vi "N-PCI6221-V02.vi"(8 "error in":errorcluster caption="错误输入", 9 "L":string, 10 "H":string, 11 "Input":string) -> (0 "error out":errorcluster caption="错误输出", 2 "布尔":bool, 3 "Output":string)   [LabVIEW 2014]
uses:
  <vilib>/DAQmx/create/channels.llb/DAQmx Create Channel (DO-Digital Output).vi
  <vilib>/DAQmx/write.llb/DAQmx Write (Digital 1D Bool 1Chan 1Samp).vi
  <vilib>/DAQmx/create/channels.llb/DAQmx Create Channel (DI-Digital Input).vi
  <vilib>/DAQmx/read.llb/DAQmx Read (Digital U8 1Chan 1Samp).vi
  <vilib>/DAQmx/read.llb/DAQmx Read (Digital Bool 1Line 1Point).vi
  <vilib>/DAQmx/write.llb/DAQmx Write (Digital 1D Bool NChan 1Samp 1Line).vi
  <vilib>/DAQmx/create/channels.llb/DAQmx Create Channel (AI-Voltage-Basic).vi
  <vilib>/DAQmx/read.llb/DAQmx Read (Analog 1D DBL 1Chan NSamp).vi
  <vilib>/DAQmx/read.llb/DAQmx Read (Analog DBL 1Chan 1Samp).vi
  <vilib>/DAQmx/configure/timing.llb/DAQmx Timing (Sample Clock).vi
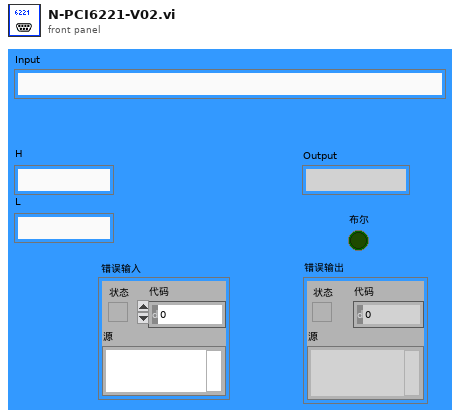
[diagram p1: front panel]
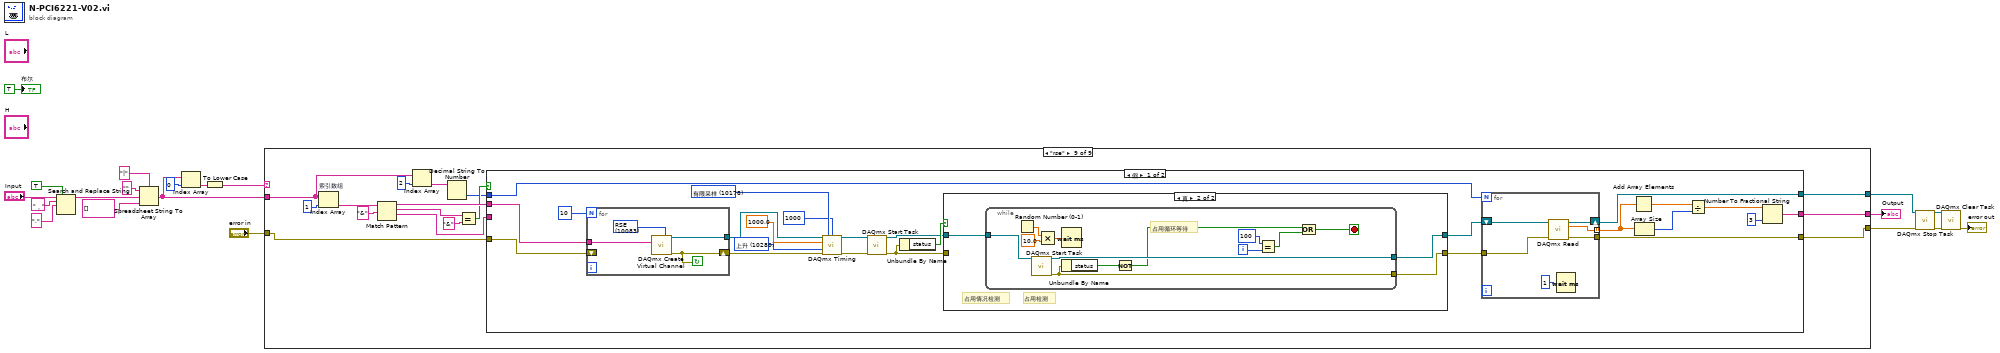
[diagram p0: block diagram]
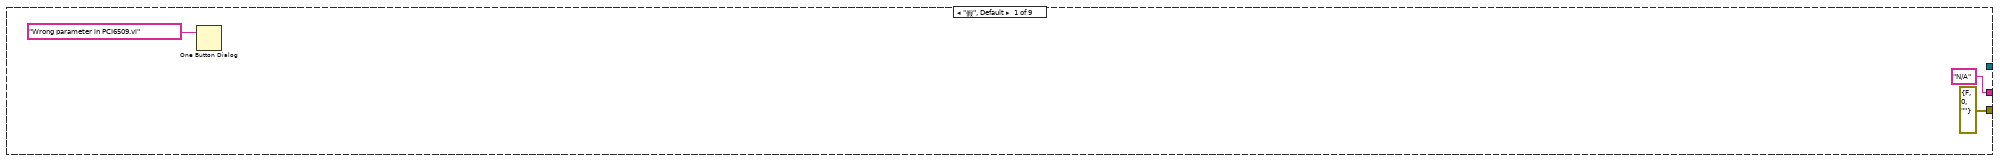
[diagram p2: hidden frame]
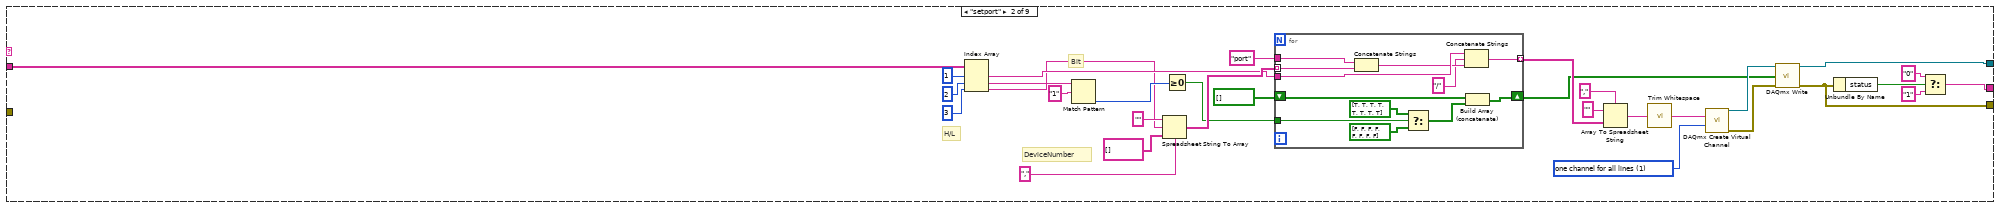
[diagram p3: hidden frame]
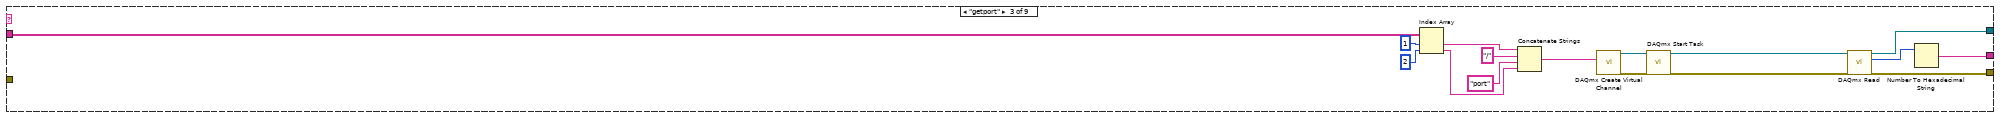
[diagram p4: hidden frame]
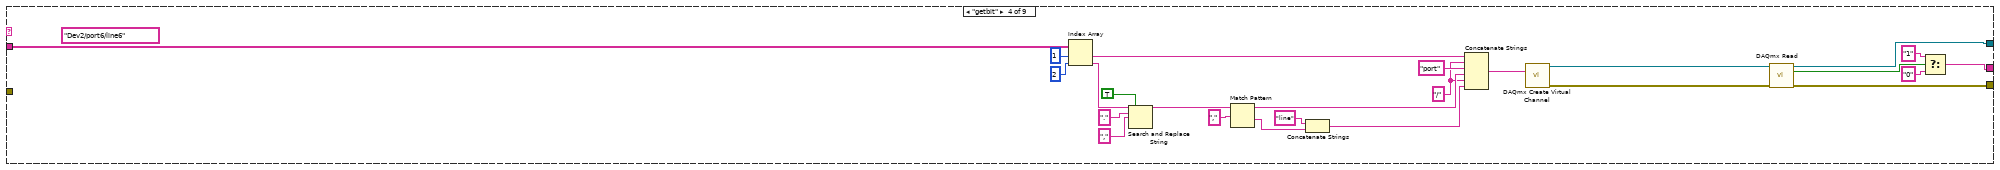
[diagram p5: hidden frame]
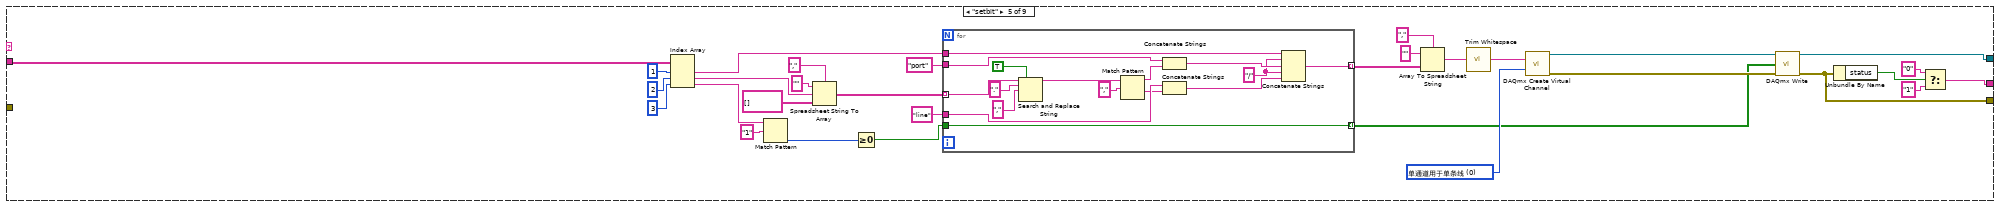
[diagram p6: hidden frame]
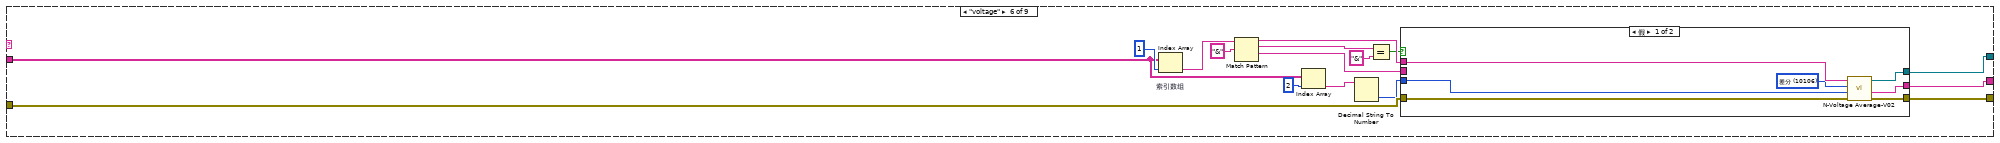
[diagram p7: hidden frame]
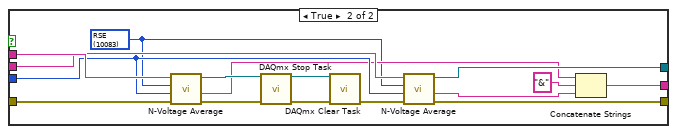
[diagram p8: hidden frame]
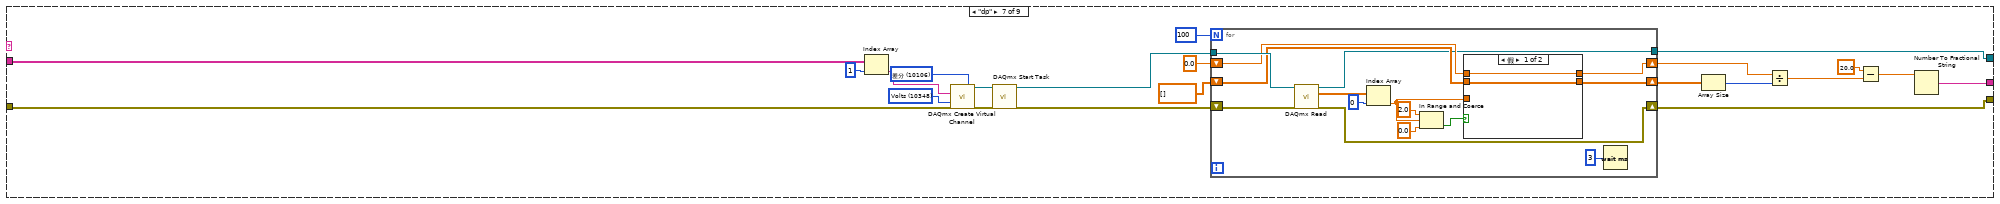
[diagram p9: hidden frame]
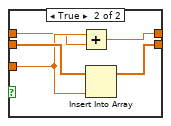
[diagram p10: hidden frame]
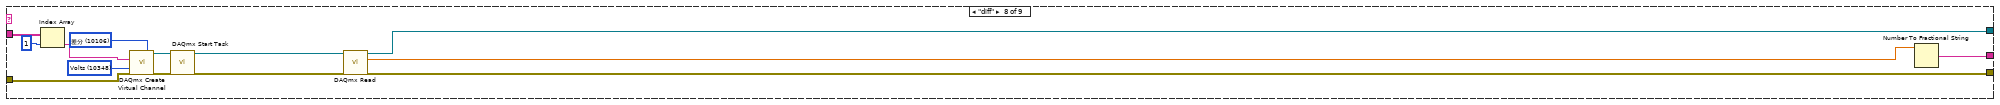
[diagram p11: hidden frame]
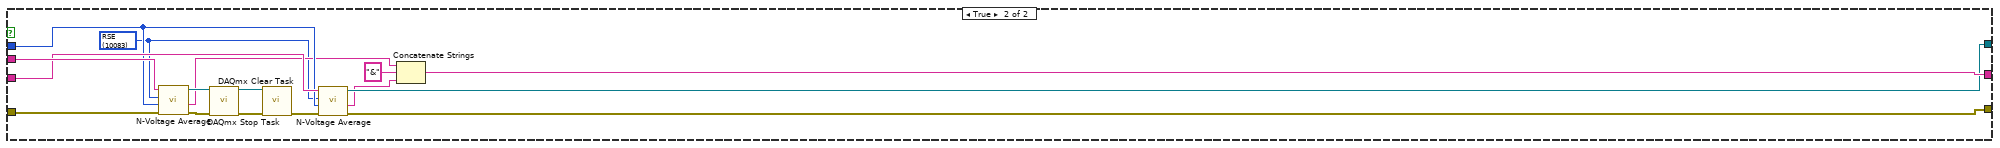
[diagram p13: hidden frame]
diagram:
  n1 = Search and Replace String(replace all?=TRUE ("替换全部？(F)"), input string="Input", search string="，" ("搜索字符串"), replace string="," ("替换字符串(\"\")")) -> (result string=w4:string)  [unwired: 4 in, 3 out]
  n2 = Spreadsheet String To Array(delimiter (Tab)="|" ("分隔符(Tab)"), format string="" ("格式字符串"), spreadsheet string=w4, array type (2D Dbl)=string[] []) -> (array=w2:string[])
  n3 = Index Array(array=w2, index=0 ("索引")) -> (element=w16:string)
  n4 = To Lower Case(string=w16) -> (all lower case string=w15:string)
  n5 = case shown="\"rse\"" w15 {
    tunnel: w2 -> [_ w31 w70 w87 w138 w157 w210 w246 w256]
    tunnel: [_ w29 w67 w85 w115 w168 w199 w241 w253] -> w14
    tunnel: [errorcluster {"status"=FALSE, "code"=0, "source"=""} ("error out") w28 w68 w86 w114 w169 w200 w242 w254] -> w13
    tunnel: ["N/A" w24 w69 w84 w110 w166 w201 w243 w255] -> w9
    tunnel: "error in" -> [_ _ _ _ _ w170 w197 w239 w257]
    frame "假", Default {
      n6 = One Button Dialog(message="Wrong parameter in PCI6509.vi") -> ()  [unwired: 2 out]
    }
    frame "setport" {
      w49 = 1 items=["one channel for each line", "one channel for all lines"] ("line grouping")
      # "H/L"
      # "Bit"
      # "DeviceNumber"
      n7 = Index Array(array=w31, index #1=1 ("index"), index #2=2 ("index"), index #3=3 ("index")) -> (element #1=w41:string, element #2=w30:string, element #3=w40:string)
      n8 = Match Pattern(string=w40, regular expression="1") -> (offset past match=w48:i32)  [unwired: 4 out]
      n9 = Spreadsheet String To Array(delimiter (Tab)=",", format string="", spreadsheet string=w30, array type (2D Dbl)=string[] []) -> (array=w45:string[])
      n10 = Greater Or Equal To 0?(x=w48) -> (x >= 0?=w35:bool)
      n11 = for {
        tunnel: w45 -> [w61] mode=indexing
        tunnel: w41 -> [w66]
        tunnel: "port" ("delimiter (Tab)") -> [w65]
        tunnel: [w62] -> w36 mode=indexing
        tunnel: w35 -> [w60]
        shift-right: [w55] -> w33
        shift-left: bool[] [] -> [w57]
        n12 = Concatenate Strings(w65, w61) -> (w64:string)
        n13 = Select(t=bool[] [TRUE, TRUE, TRUE, TRUE, TRUE, TRUE, TRUE, TRUE], s=w60, f=bool[] [FALSE, FALSE, FALSE, FALSE, FALSE, FALSE, FALSE, FALSE]) -> (s? t:f=w56:bool[])
        n14 = Concatenate Strings(w66, "/" ("delimiter (Tab)"), w64) -> (w62:string)
        n15 = Build Array (concatenate)(w57, w56) -> (w55:bool[])
      }
      n16 = Array To Spreadsheet String(delimiter (Tab)=",", array=w36, 3:"" ("format string")) -> (spreadsheet string=w37:string)
      n17 = call <vilib>:"Trim Whitespace.vi"("string"=w37) -> ("trimmed string"=w32:string)  [unwired: 1 in]
      n18 = call-poly <vilib>:"DAQmx Create Virtual Channel.vi"("lines"=w32, "line grouping"=w49) -> ("task out"=w50:refnum<k21>, "error out"=w51:errorcluster)  [unwired: 3 in, 9 out]
      n19 = call-poly <vilib>:"DAQmx Write.vi"("task/channels in"=w50, "data"=w33, "error in"=w51) -> ("task out"=w29:refnum<k21>, "error out"=w28:errorcluster)  [unwired: 1 in, 10 out]
      n20 = Unbundle By Name(w28) -> ("status"=w27:bool)
      n21 = Select(t="0", s=w27, f="1") -> (s? t:f=w24:string)
    }
    frame "getport" {
      n22 = Index Array(array=w70, index #1=1 ("index"), index #2=2 ("index")) -> (element #1=w80:string, element #2=w77:string)
      n23 = Concatenate Strings(w80, "/" ("string"), "port" ("string"), w77) -> (w76:string)
      n24 = call-poly <vilib>:"DAQmx Create Virtual Channel.vi"("lines"=w76) -> ("task out"=w74:refnum<k21>, "error out"=w71:errorcluster)  [unwired: 4 in, 9 out]
      n25 = call <vilib>:"DAQmx Start Task.vi"("task/channels in"=w74, "error in"=w71) -> ("task out"=w73:refnum<k21>, "error out"=w72:errorcluster)  [unwired: 12 out]
      n26 = call-poly <vilib>:"DAQmx Read.vi"("task/channels in"=w73, "error in"=w72) -> ("task out"=w67:refnum<k21>, "data"=w75:u8, "error out"=w68:errorcluster)  [unwired: 11 out]
      n27 = Number To Hexadecimal String(2:w75) -> (0:w69:string)  [unwired: 1 out]
    }
    frame "getbit" {
      (unwired) tag "Dev2/port6/line6" ("lines")
      w94 = "/" ("string")
      n28 = Index Array(array=w87, index #1=1 ("index"), index #2=2 ("index")) -> (element #1=w103:string, element #2=w100:string)
      n29 = Search and Replace String(replace all?=TRUE ("replace all? (F)"), input string=w100, search string=".", replace string="," ("replace string (\"\")")) -> (result string=w97:string)  [unwired: 1 in, 6 out]
      n30 = Match Pattern(string=w97, regular expression=",") -> (before substring=w95:string, after substring=w92:string)  [unwired: 3 out]
      n31 = Concatenate Strings("line" ("string"), w92) -> (w91:string)
      n32 = Concatenate Strings(w103, w94, "port" ("string"), w95, w94, w91) -> (w90:string)
      n33 = call-poly <vilib>:"DAQmx Create Virtual Channel.vi"("lines"=w90) -> ("task out"=w105:refnum<k21>, "error out"=w104:errorcluster)  [unwired: 4 in, 9 out]
      n34 = call-poly <vilib>:"DAQmx Read.vi"("task/channels in"=w105, "error in"=w104) -> ("task out"=w85:refnum<k21>, "data"=w83:bool, "error out"=w86:errorcluster)  [unwired: 11 out]
      n35 = Select(t="1", s=w83, f="0") -> (s? t:f=w84:string)
    }
    frame "setbit" {
      w119 = 0 items=["单通道用于单条线", "单通道用于所有线"] ("line grouping")
      n36 = Index Array(array=w138, index #1=1 ("索引"), index #2=2 ("索引"), index #3=3 ("索引")) -> (element #1=w129:string, element #2=w135:string, element #3=w126:string)
      n37 = Match Pattern(string=w126, regular expression="1" ("正则表达式")) -> (offset past match=w124:i32)  [unwired: 4 out]
      n38 = Spreadsheet String To Array(delimiter (Tab)="," ("分隔符(Tab)"), format string="" ("格式字符串"), spreadsheet string=w135, array type (2D Dbl)=string[] []) -> (array=w128:string[])
      n39 = Greater Or Equal To 0?(x=w124) -> (x >= 0?=w123:bool)
      n40 = for {
        tunnel: w128 -> [w141] mode=indexing
        tunnel: w129 -> [w153]
        tunnel: "port" ("格式字符串") -> [w152]
        tunnel: "line" ("格式字符串") -> [w150]
        tunnel: [w145] -> w122 mode=indexing
        tunnel: w123 -> [w139]
        tunnel: [w139] -> w116 mode=indexing
        w147 = "/" ("delimiter (Tab)")
        n41 = Search and Replace String(replace all?=TRUE ("replace all? (F)"), input string=w141, search string=".", replace string="," ("replace string (\"\")")) -> (result string=w140:string)  [unwired: 1 in, 6 out]
        n42 = Match Pattern(string=w140, regular expression=",") -> (before substring=w151:string, after substring=w149:string)  [unwired: 3 out]
        n43 = Concatenate Strings(w152, w151) -> (w148:string)
        n44 = Concatenate Strings(w150, w149) -> (w146:string)
        n45 = Concatenate Strings(w153, w147, w148, w147, w146) -> (w145:string)
      }
      n46 = Array To Spreadsheet String(delimiter (Tab)="," ("分隔符(Tab)"), array=w122, 3:"" ("格式字符串")) -> (spreadsheet string=w109:string)
      n47 = call <vilib>:"Trim Whitespace.vi"("string"=w109) -> ("trimmed string"=w108:string)  [unwired: 1 in]
      n48 = call-poly <vilib>:"DAQmx Create Virtual Channel.vi"("lines"=w108, "line grouping"=w119) -> ("task out"=w118:refnum<k21>, "error out"=w117:errorcluster)  [unwired: 3 in, 9 out]
      n49 = call-poly <vilib>:"DAQmx Write.vi"("task/channels in"=w118, "data"=w116, "error in"=w117) -> ("task out"=w115:refnum<k21>, "error out"=w114:errorcluster)  [unwired: 1 in, 10 out]
      n50 = Unbundle By Name(w114) -> ("status"=w113:bool)
      n51 = Select(t="0", s=w113, f="1") -> (s? t:f=w110:string)
    }
    frame "voltage" {
      n52 = Index Array "索引数组"(array=w157, index=1) -> (element=w165:string)
      n53 = Match Pattern(string=w165, regular expression="&" ("正则表达式")) -> (before substring=w161:string, match substring=w163:string, after substring=w160:string)  [unwired: 1 in, 1 out]
      n54 = Index Array(array=w157, index=2) -> (element=w156:string)
      n55 = Decimal String To Number(string=w156) -> (number=w155:i32)  [unwired: 2 in, 1 out]
      n56 = Equal?(x=w163, y="&" ("正则表达式")) -> (x = y?=w159:bool)
      n57 = case shown="假" w159 {
        tunnel: w170 -> [w176 w193]
        tunnel: [w175 w183] -> w169
        tunnel: [w174 w182] -> w168
        tunnel: [w173 w184] -> w166
        tunnel: w161 -> [w177 w187]
        tunnel: w160 -> [_ w186]
        tunnel: w155 -> [w172 w181]
        frame False {
          w171 = 10106 items=["默认"=-1, "RSE"=10083, "NRSE"=10078, "差分"=10106, "伪差分"=12529] ("Type")
          n58 = call "N-Voltage Average-V02.vi"("error in"=w176, "Times"=w172, "Type"=w171, "Channel"=w177) -> ("error out"=w175:errorcluster, "Voltage"=w173:string, "task out"=w174:refnum<k21>)  [unwired: 1 in]
        }
        frame True {
          w178 = 10083 items=["默认"=-1, "RSE"=10083, "NRSE"=10078, "差分"=10106, "伪差分"=12529] ("Type")
          n59 = call "N-Voltage Average.vi"("error in"=w193, "Times"=w181, "Type"=w178, "Channel"=w187) -> ("error out"=w189:errorcluster, "Voltage"=w180:string, "task out"=w190:refnum<k21>)  [unwired: 1 in]
          n60 = call <vilib>:"DAQmx Stop Task.vi"("task/channels in"=w190, "error in"=w189) -> ("task out"=w191:refnum<k21>, "error out"=w192:errorcluster)  [unwired: 12 out]
          n61 = call <vilib>:"DAQmx Clear Task.vi"("task in"=w191, "error in"=w192) -> ("error out"=w188:errorcluster)  [unwired: 13 out]
          n62 = call "N-Voltage Average.vi"("error in"=w188, "Times"=w181, "Type"=w178, "Channel"=w186) -> ("error out"=w183:errorcluster, "Voltage"=w179:string, "task out"=w182:refnum<k21>)  [unwired: 1 in]
          n63 = Concatenate Strings(w180, "&" ("字符串"), w179) -> (w184:string)
        }
      }
    }
    frame "dp" {
      w212 = 10348 items=["Volts"=10348, "来自自定义换算"=10065] ("units")
      w215 = 10106 items=["默认"=-1, "RSE"=10083, "NRSE"=10078, "差分"=10106, "伪差分"=12529] ("input terminal configuration")
      n64 = Index Array(array=w210, index=1) -> (element=w209:string)
      n65 = call-poly <vilib>:"DAQmx Create Virtual Channel.vi"("input terminal configuration"=w215, "physical channels"=w209, "units"=w212, "error in"=w197) -> ("task out"=w213:refnum<k21>, "error out"=w214:errorcluster)  [unwired: 5 in, 5 out]
      n66 = call <vilib>:"DAQmx Start Task.vi"("task/channels in"=w213, "error in"=w214) -> ("task out"=w207:refnum<k21>, "error out"=w198:errorcluster)  [unwired: 12 out]
      n67 = for {
        N: 100 -> [_]
        tunnel: w207 -> [w230]
        shift-right: [w222] -> w205
        shift-left: dbl[] [] -> [w224]
        shift-right: [w220] -> w202
        shift-left: 0.0 ("下限") -> [w221]
        tunnel: [w218] -> w199
        shift-right: [w219] -> w200
        shift-left: w198 -> [w217]
        n68 = call-poly <vilib>:"DAQmx Read.vi"("task/channels in"=w230, "error in"=w217) -> ("task out"=w218:refnum<k21>, "data"=w229:dbl[], "error out"=w219:errorcluster)  [unwired: 1 in, 10 out]
        n69 = Index Array(array=w229, index=0 ("索引")) -> (element=w223:dbl)
        n70 = In Range and Coerce(upper limit=2.0 ("上限"), x=w223, lower limit=0.0 ("下限")) -> (In Range?=w225:bool)  [unwired: 1 out]
        n71 = case shown="假" w225 {
          tunnel: w224 -> [w232 w237]
          tunnel: w223 -> [_ w235]
          tunnel: [w232 w236] -> w222
          tunnel: w221 -> [w231 w234]
          tunnel: [w231 w233] -> w220
          frame False {
          }
          frame True {
            n72 = Add(x=w235, y=w234) -> (x+y=w233:dbl)
            n73 = Insert Into Array(array=w237, new element=w235) -> (w236:dbl[])  [unwired: 1 in]
          }
        }
        n74 = Wait (ms)(milliseconds to wait=u32 3 ("等待时间（毫秒）")) -> ()  [unwired: 1 out]
      }
      n75 = Array Size(array=w205) -> (size(s)=w203:i32)
      n76 = Divide(x=w202, y=w203) -> (x/y=w195:dbl)
      n77 = Subtract(x=20.0 ("下限"), y=w195) -> (x-y=w194:dbl)
      n78 = Number To Fractional String(number=w194) -> (F-format string=w201:string)  [unwired: 3 in]
    }
    frame "diff" {
      w248 = 10348 items=["Volts"=10348, "来自自定义换算"=10065] ("units")
      w251 = 10106 items=["默认"=-1, "RSE"=10083, "NRSE"=10078, "差分"=10106, "伪差分"=12529] ("input terminal configuration")
      n79 = Index Array(array=w246, index=1) -> (element=w245:string)
      n80 = call-poly <vilib>:"DAQmx Create Virtual Channel.vi"("input terminal configuration"=w251, "physical channels"=w245, "units"=w248, "error in"=w239) -> ("task out"=w249:refnum<k21>, "error out"=w250:errorcluster)  [unwired: 5 in, 5 out]
      n81 = call <vilib>:"DAQmx Start Task.vi"("task/channels in"=w249, "error in"=w250) -> ("task out"=w244:refnum<k21>, "error out"=w240:errorcluster)  [unwired: 12 out]
      n82 = call-poly <vilib>:"DAQmx Read.vi"("task/channels in"=w244, "error in"=w240) -> ("task out"=w241:refnum<k21>, "data"=w238:dbl, "error out"=w242:errorcluster)  [unwired: 11 out]
      n83 = Number To Fractional String(number=w238) -> (F-format string=w243:string)  [unwired: 3 in]
    }
    frame "rse" {
      n84 = Index Array "索引数组"(array=w256, index=1) -> (element=w252:string)
      n85 = Match Pattern(string=w252, regular expression="&" ("正则表达式")) -> (before substring=w263:string, match substring=w265:string, after substring=w262:string)  [unwired: 1 in, 1 out]
      n86 = Index Array(array=w256, index=2) -> (element=w259:string)
      n87 = Decimal String To Number(string=w259) -> (number=w258:i32)  [unwired: 2 in, 1 out]
      n88 = Equal?(x=w265, y="&" ("正则表达式")) -> (x = y?=w261:bool)
      n89 = case shown="假" w261 {
        tunnel: w257 -> [w291 w335]
        tunnel: [w287 w325] -> w254
        tunnel: [w288 w324] -> w253
        tunnel: [w289 w326] -> w255
        tunnel: w263 -> [w292 w329]
        tunnel: w262 -> [_ w328]
        tunnel: w258 -> [w290 w323]
        frame False {
          w283 = 10178 items=["有限采样"=10178, "连续采样"=10123, "硬件定时单点"=12522] ("sample mode")
          w284 = 10280 items=["上升"=10280, "下降"=10171] ("active edge")
          n90 = for {
            N: 10 -> [_]
            tunnel: w292 -> [w312]
            tunnel: [w311] -> w279
            shift-right: [w310] -> w278
            shift-left: w291 -> [_]
            stop <- w310 continue-if-true
            w313 = 10083 items=["默认"=-1, "RSE"=10083, "NRSE"=10078, "差分"=10106, "伪差分"=12529] ("Type")
            n91 = call-poly <vilib>:"DAQmx Create Virtual Channel.vi"("input terminal configuration"=w313, "physical channels"=w312) -> ("task out"=w311:refnum<k21>, "error out"=w310:errorcluster)  [unwired: 12 in]
          }
          n92 = call-poly <vilib>:"DAQmx Timing.vi"("task/channels in"=w279, "sample mode"=w283, "samples per channel"=1000, "rate"=1000.0, "active edge"=w284, "error in"=w278) -> ("task out"=w280:refnum<k21>, "error out"=w281:errorcluster)  [unwired: 8 in]
          n93 = call <vilib>:"DAQmx Start Task.vi"("task/channels in"=w280, "error in"=w281) -> ("task out"=w271:refnum<k21>, "error out"=w268:errorcluster)  [unwired: 12 in]
          n94 = Unbundle By Name(w268) -> ("status"=w272:bool)
          n95 = case shown="真" w272 {
            tunnel: [w293 w297] -> w270
            tunnel: [w294 w296] -> w269
            tunnel: w271 -> [w293 w295]
            tunnel: w268 -> [w294 _]
            frame False {
            }
            frame True {
              # "占用检测"
              # "占用情况检测"
              n96 = while {
                tunnel: [w309] -> w297
                tunnel: [w302] -> w296
                tunnel: w295 -> [w301]
                i -> [w308]
                stop <- w306 stop-if-true
                # "占用循环等待"
                n97 = Random Number (0-1)() -> (number: 0 to 1=w300:dbl)
                n98 = call <vilib>:"DAQmx Start Task.vi"("task/channels in"=w301) -> ("task out"=w309:refnum<k21>, "error out"=w302:errorcluster)  [unwired: 13 in]
                n99 = Multiply(x=w300, y=10.0) -> (x*y=w298:dbl)
                n100 = Wait (ms)(milliseconds to wait=w298) -> ()  [unwired: 1 out]
                n101 = Unbundle By Name(w302) -> ("status"=w304:bool)
                n102 = Not(x=w304) -> (.not. x?=w303:bool)
                n103 = Equal?(x=100, y=w308) -> (x = y?=w305:bool)
                n104 = Or(x=w303, y=w305) -> (x .or. y?=w306:bool)
              }
            }
          }
          n105 = for {
            N: w290 -> [_]
            tunnel: w269 -> [w319]
            tunnel: [w318] -> w287
            tunnel: [w314] -> w277 mode=indexing
            shift-right: [w317] -> w288
            shift-left: w270 -> [w316]
            n106 = call-poly <vilib>:"DAQmx Read.vi"("task/channels in"=w316, "error in"=w319) -> ("task out"=w317:refnum<k21>, "data"=w314:dbl, "error out"=w318:errorcluster)  [unwired: 11 in]
            n107 = Wait (ms)(milliseconds to wait=u32 1 ("等待时间（毫秒）")) -> ()  [unwired: 1 out]
          }
          n108 = Add Array Elements(numeric array=w277) -> (sum=w276:dbl)
          n109 = Array Size(array=w277) -> (size(s)=w275:i32)
          n110 = Divide(x=w276, y=w275) -> (x/y=w274:dbl)
          n111 = Number To Fractional String(number=w274, precision (6)=i16 3 ("精度(6)")) -> (F-format string=w289:string)  [unwired: 2 in]
        }
        frame True {
          w320 = 10083 items=["默认"=-1, "RSE"=10083, "NRSE"=10078, "差分"=10106, "伪差分"=12529] ("Type")
          n112 = call "N-Voltage Average.vi"("error in"=w335, "Times"=w323, "Type"=w320, "Channel"=w329) -> ("error out"=w331:errorcluster, "Voltage"=w322:string, "task out"=w332:refnum<k21>)  [unwired: 1 in]
          n113 = call <vilib>:"DAQmx Stop Task.vi"("task/channels in"=w332, "error in"=w331) -> ("task out"=w333:refnum<k21>, "error out"=w334:errorcluster)  [unwired: 12 out]
          n114 = call <vilib>:"DAQmx Clear Task.vi"("task in"=w333, "error in"=w334) -> ("error out"=w330:errorcluster)  [unwired: 13 out]
          n115 = call "N-Voltage Average.vi"("error in"=w330, "Times"=w323, "Type"=w320, "Channel"=w328) -> ("error out"=w325:errorcluster, "Voltage"=w321:string, "task out"=w324:refnum<k21>)  [unwired: 1 in]
          n116 = Concatenate Strings(w322, "&" ("字符串"), w321) -> (w326:string)
        }
      }
    }
  }
  "Output" <- w9
  n117 = call <vilib>:"DAQmx Stop Task.vi"("task/channels in"=w14, "error in"=w13) -> ("task out"=w12:refnum<k21>, "error out"=w11:errorcluster)  [unwired: 12 out]
  n118 = call <vilib>:"DAQmx Clear Task.vi"("task in"=w12, "error in"=w11) -> ("error out"=→"error out":errorcluster)  [unwired: 13 out]
  "布尔" <- TRUE ("布尔")
